vi "移动平均值.vi"() -> ()   [LabVIEW 2014]
panel:
  out "循环次数":i32
  out "移动平均值":dbl
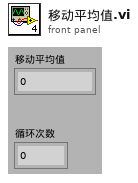
[diagram p1: front panel]
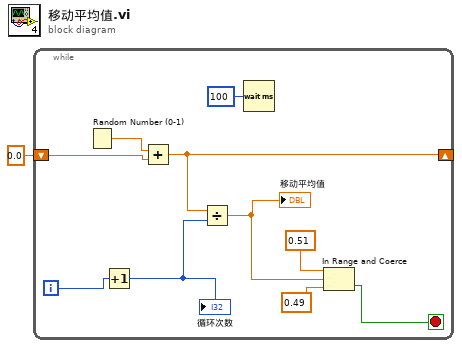
[diagram p0: block diagram]
diagram:
  n1 = while {
    shift-right: [w9] -> _
    shift-left: 0.0 -> [w10]
    i -> [w8]
    stop <- w3 stop-if-true
    n2 = Random Number (0-1)() -> (number: 0 to 1=w11:dbl)
    n3 = Increment(x=w8) -> (x+1=w7:i32)
    "循环次数" <- w7
    n4 = Add(x=w11, y=w10) -> (x+y=w9:dbl)
    n5 = Divide(x=w9, y=w7) -> (x/y=w6:dbl)
    "移动平均值" <- w6
    n6 = Wait (ms)(milliseconds to wait=u32 100 ("等待时间（毫秒）")) -> ()  [unwired: 1 out]
    n7 = In Range and Coerce(upper limit=0.51 ("上限"), x=w6, lower limit=0.49 ("下限")) -> (In Range?=w3:bool)  [unwired: 1 out]
  }
